vi "FileIO-List Parameter Files Heirarchically.vi"(7 "folder":path, 11 "error in (no error)":errorcluster) -> (8 "Parameter file names":string[](array[string]))   [LabVIEW 2020]
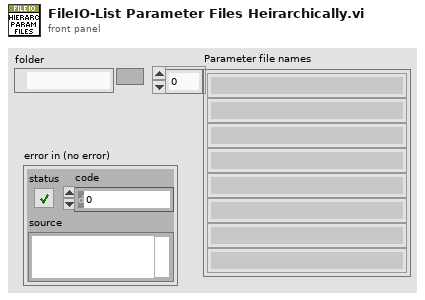
[diagram p1: front panel]
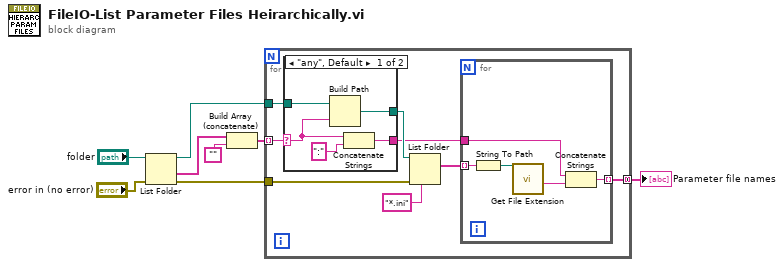
[diagram p0: block diagram]
diagram:
  n1 = List Folder(path="folder", error in="error in (no error)") -> (path out=w2:path, folder names=w5:string[], error out=w1:errorcluster)  [unwired: 2 in, 1 out]
  n2 = Build Array (concatenate)(w5, "") -> (w3:string[])
  n3 = for {
    tunnel: [w16] -> w7 mode=concatenating
    tunnel: w3 -> [w10] mode=indexing
    tunnel: w2 -> [w15]
    tunnel: w1 -> [w11]
    n4 = case shown="\"any\", Default" w10 {
      selector: w10 -> [w18 w22]
      tunnel: w15 -> [w21 w23]
      tunnel: [w20 w23] -> w14
      tunnel: [w19 w22] -> w9
      frame "any", Default {
        n5 = Build Path(base path=w21, name or relative path=w18) -> (appended path=w20:path)
        n6 = Concatenate Strings(w18, ":" ("string")) -> (w19:string)
      }
      frame "" {
      }
    }
    n7 = List Folder(path=w14, pattern="*.ini", error in=w11) -> (filenames=w13:string[])  [unwired: 1 in, 3 out]
    n8 = for {
      tunnel: w13 -> [w27] mode=indexing
      tunnel: [w25] -> w16 mode=indexing
      tunnel: w9 -> [w24]
      n9 = String To Path(string=w27) -> (path=w28:path)
      n10 = call <vilib>:"Get File Extension.vi"("file"=w28) -> ("filename without extension"=w26:string)  [unwired: 6 in, 4 out]
      n11 = Concatenate Strings(w24, w26) -> (w25:string)
    }
  }
  "Parameter file names" <- w7
